vi "WPI_CameraGet Image From Controller.vi"(4 "Camera Settings":T3={"name"="", "fps"=30, "compression"=30, "Image Size"=enum."320x240"}, 5 "parameters":T1(array[cluster]), 6 "cgi String":string, 7 "port":u16=1180, 8 "error in (no error)":errorcluster, 9 "Operation":enum16{"Read", "Reopen", "Close"}(ring), 10 "Controller Address":string, 11 "Image":T4) -> (0 "error out":errorcluster, 2 "Bandwidth (Mbps)":dbl=30.0, 3 "Image Out":T4(plugin-control))   [LabVIEW 2017]
doc: "Retrieves a specific image from the image data that the camera connected to the CompactRIO device you specify acquired. Use this VI in the FRC dashboard project on the host computer.\n\nThis software is licensed. Open the labview\\readme\\WPI Robotics Library Open Source License.txt file for more information."
uses:
  <vilib>/vision/Image Controls.llb/IMAQ Image.ctl
  <vilib>/Rock Robotics/WPI/Camera/WPI_CameraImageSize.ctl
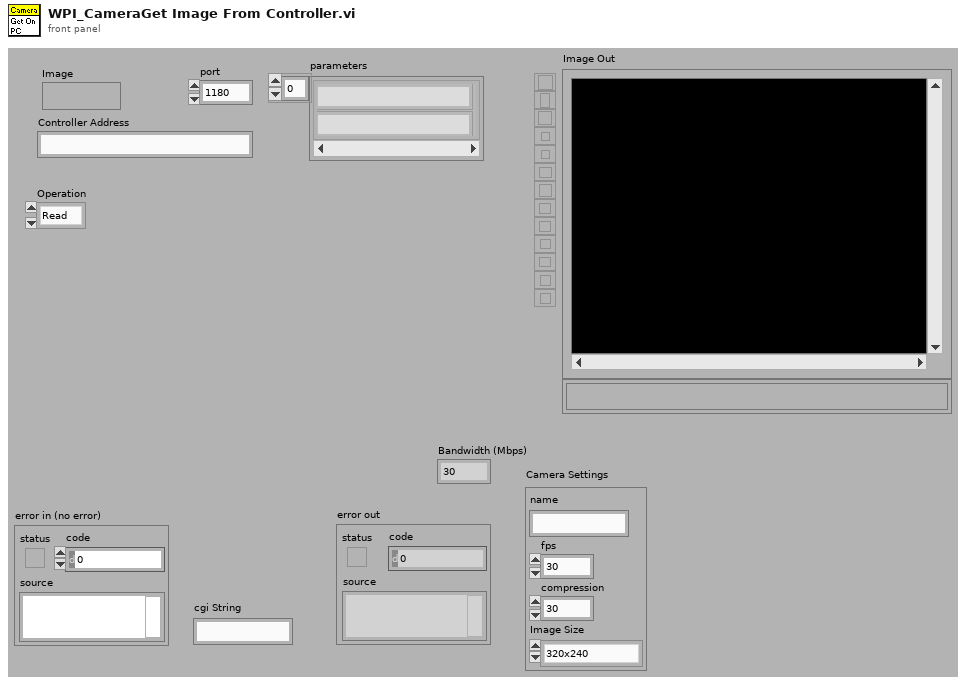
[diagram p1: front panel]
types:
  T1 = cluster{"token string":string, "token string 2":string}[]
  T2 = typedef "WPI_CameraImageSize.ctl" = enum16{"640x480", "320x240", "160x120", "Custom"}
  T3 = cluster{"name":string, "fps":i32, "compression":i32, "Image Size":T2}
  T4 = typedef "IMAQ Image.ctl" = refnum<image>
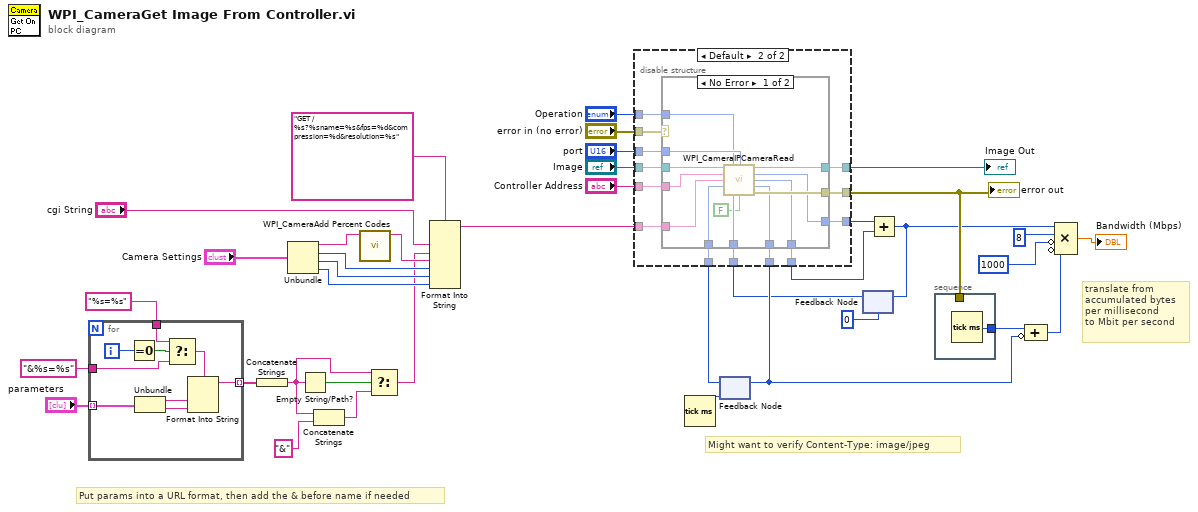
[diagram p0: block diagram]
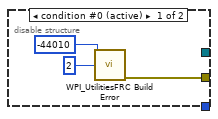
[diagram p2: hidden frame]
diagram:
  # "Put params into a URL format, then add the & before name if needed"
  # "Might want to verify Content-Type: image/jpeg"
  # "translate from\naccumulated bytes\nper millisecond \nto Mbit per second"
  n1 = for {
    tunnel: "parameters" -> [w47] mode=indexing
    tunnel: "%s=%s" -> [w41]
    tunnel: [w40] -> w9 mode=indexing
    tunnel: "&%s=%s" -> [w39]
    i -> [w43]
    n2 = Equal To 0?(x=w43) -> (x = 0?=w44:bool)
    n3 = Unbundle(w47) -> ("token string"=w46:string, "token string 2"=w45:string)
    n4 = Select(t=w41, s=w44, f=w39) -> (s? t:f=w42:string)
    n5 = Format Into String(format string=w42, w46, w45) -> (resulting string=w40:string)  [unwired: 2 in, 1 out]
  }
  n6 = Concatenate Strings(w9) -> (w5:string)
  n7 = Unbundle("Camera Settings") -> ("name"=w14:string, "fps"=w17:i32, "compression"=w16:i32, "Image Size"=w15:T2)
  n8 = Empty String/Path?(string/path=w5) -> (empty?=w8:bool)
  n9 = Concatenate Strings(w5, "&") -> (w3:string)
  n10 = call <vilib>:"WPI_CameraAdd Percent Codes.vi"("String"=w14) -> ("String 2"=w13:string)  [unwired: 10 in]
  n11 = Select(t=w5, s=w8, f=w3) -> (s? t:f=w6:string)
  n12 = Format Into String(format string="GET /%s?%sname=%s&fps=%d&compression=%d&resolution=%s", "cgi String", w6, w13, w17, w16, w15) -> (resulting string=w2:string)  [unwired: 2 in, 1 out]
  n13 = Tick Count (ms)() -> (millisecond timer value=w34:u32)
  n14 = feedback #1(w34) -> (w24:u32)
  n15 = feedback #2(0) -> (w23:i32)
  n16 = disable-structure shown="Default" {
    disable-tunnel: "error in (no error)" -> [_ w63]
    disable-tunnel: [w48 w62] -> w27
    disable-tunnel: "Image" -> [_ w61]
    disable-tunnel: [_ w60] -> w36
    disable-tunnel: "Controller Address" -> [_ w59]
    disable-tunnel: [_ w58] -> w25
    disable-tunnel: w24 -> [_ w57]
    disable-tunnel: w23 -> [_ w56]
    disable-tunnel: [_ w55] -> w22
    disable-tunnel: [_ w54] -> w21
    disable-tunnel: "port" -> [_ w53]
    disable-tunnel: w2 -> [_ w52]
    disable-tunnel: "Operation" -> [_ w51]
    frame condition #0 (active) {
      n17 = call <vilib>:"WPI_UtilitiesFRC Build Error.vi"("error code"=-44010 ("code"), "chain levels to remove (1)"=2) -> ("error out"=w48:errorcluster)  [unwired: 3 in, 10 out]
    }
    frame condition #1 {
      n18 = case shown="No Error" w63 {
        selector: w63 -> [_ w77]
        tunnel: [w76 w77] -> w62
        tunnel: w61 -> [w75 w78]
        tunnel: [w74 w78] -> w60
        tunnel: w59 -> [w73 _]
        tunnel: [w72 w80] -> w58
        tunnel: w57 -> [w71 w80]
        tunnel: w56 -> [w70 w79]
        tunnel: [w69 w79] -> w55
        tunnel: [w68 _] -> w54
        tunnel: w53 -> [w67 _]
        tunnel: w52 -> [w66 _]
        tunnel: w51 -> [w64 _]
        frame No Error {
          n19 = call <vilib>:"WPI_CameraIPCameraRead.vi"("Refnum in"=w75, "Operation"=w64, "port"=w67, "address"=w73, "cgi string"=w66, "millisecs in"=w71, "accum length in"=w70, "Authenticate"=FALSE) -> ("Refnum out"=w74:T4, "length"=w68:i32, "accum length out"=w69:i32, "millisecs out"=w72:u32, "error out"=w76:errorcluster)  [unwired: 3 in]
        }
        frame Error {
        }
      }
    }
  }
  "error out" <- w27
  "Image Out" <- w36
  n20 = feedback-in #1(w25) -> ()
  n21 = Add(x=w21, y=w22) -> (x+y=w26:i32)
  n22 = feedback-in #2(w26) -> ()
  n23 = stacked-sequence {
    tunnel: [w81] -> w30
    tunnel: w27 -> [_]
    frame #0 {
      n24 = Tick Count (ms)() -> (millisecond timer value=w81:u32)
    }
  }
  n25 = Compound Arithmetic op=ADD(w30, invert w25) -> (w31:u32)
  n26 = Compound Arithmetic op=MULTIPLY(w26, 8 ("timeout ms (25000)"), invert 1000 ("timeout ms (25000)"), invert w31) -> (→"Bandwidth (Mbps)":dbl)
